vi "convers.vi"(9 "Y":i32, 10 "x":i32) -> (2 "salida":string)   [LabVIEW 2016]
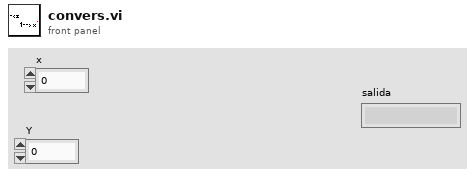
[diagram p1: front panel]
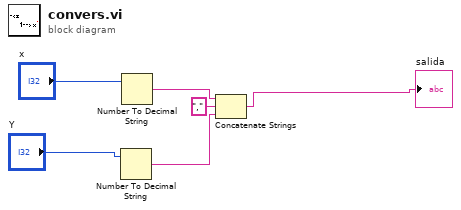
[diagram p0: block diagram]
diagram:
  n1 = Number To Decimal String(number="Y") -> (decimal integer string=w3:string)  [unwired: 1 in]
  n2 = Number To Decimal String(number="x") -> (decimal integer string=w4:string)  [unwired: 1 in]
  n3 = Concatenate Strings(w4, "," ("string"), w3) -> (→"salida":string)
